vi "Agilent VNA Set Frequency On-Off.vi"(7 "Agilent VNA":T1, 8 "error in (no error)":errorcluster, 10 "Blank Frequencies (F)":bool, 11 "VISA Resource Name":refnum<visa-resource-name>) -> (0 "error out":errorcluster, 3 "dup VISA Resource Name":refnum<visa-resource-name>)   [LabVIEW 2011]
doc: "This VI for the HP8753B Network Analyzers reads the stimulus values. Except when performing log sweeps and freq list sweeps, this VI uses the start and stop values and the number of points to calcuate the stimulus values."
uses:
  TypeDefs/Agilent VNA Instrument Info.ctl
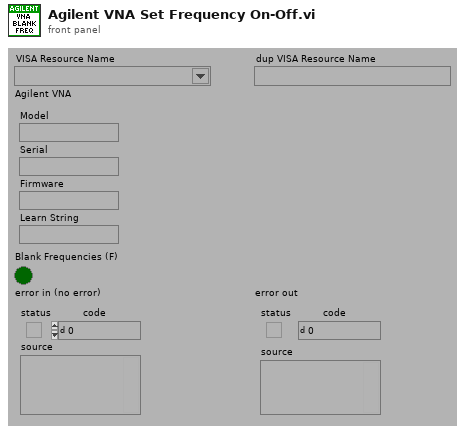
[diagram p1: front panel]
types:
  T1 = typedef "Agilent VNA Instrument Info.ctl" = cluster{"Model":string, "Serial":string, "Firmware":string, "Learn String":string}
  T2 = typedef "Agilent VNA Model.ctl" = enum16{"Not Supported", "8510X", "8719X", "8720X", "8722X", "8753X", "ENA", "PNA", "Field Fox"}
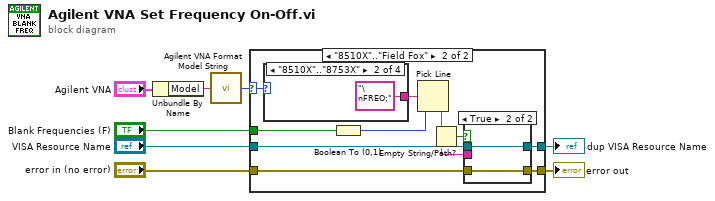
[diagram p0: block diagram]
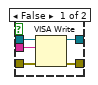
[diagram p3: hidden frame]
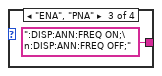
[diagram p5: hidden frame]
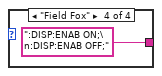
[diagram p6: hidden frame]
diagram:
  n1 = Unbundle By Name("Agilent VNA") -> ("Model"=w2:string)
  n2 = call "Agilent VNA Format Model String.vi"("Model"=w2) -> ("Model"=w1:T2)
  n3 = case shown="\"8510X\"..\"Field Fox\"" w1 {
    selector: w1 -> [_ w16]
    tunnel: [w10 w20] -> w8
    tunnel: [w9 w19] -> w7
    tunnel: "error in (no error)" -> [w9 w18]
    tunnel: "VISA Resource Name" -> [w10 w17]
    tunnel: "Blank Frequencies (F)" -> [_ w15]
    frame "Not Supported" {
    }
    frame "8510X".."Field Fox" {
      n4 = case shown="\"8510X\"..\"8753X\"" w16 {
        tunnel: [_ "\nFREO;" ":DISP:ANN:FREQ ON;\n:DISP:ANN:FREQ OFF;" ":DISP:ENAB ON;\n:DISP:ENAB OFF;"] -> w13
        frame "Not Supported" {
        }
        frame "8510X".."8753X" {
        }
        frame "ENA", "PNA" {
        }
        frame "Field Fox" {
        }
      }
      n5 = Boolean To (0,1)(Boolean=w15) -> (0, 1=w14:i16)
      n6 = Pick Line(multi-line string=w13, line index=w14) -> (output string=w12:string)  [unwired: 1 in]
      n7 = Empty String/Path?(string/path=w12) -> (empty?=w11:bool)
      n8 = case shown="True" w11 {
        tunnel: [w25 w27] -> w20
        tunnel: [w24 w26] -> w19
        tunnel: w18 -> [w23 w26]
        tunnel: w17 -> [w22 w27]
        tunnel: w12 -> [w21 _]
        frame False {
          n9 = VISA Write(VISA resource name=w22, write buffer=w21, error in (no error)=w23) -> (VISA resource name out=w25:refnum<visa-resource-name>, error out=w24:errorcluster)  [unwired: 1 out]
        }
        frame True {
        }
      }
    }
  }
  "dup VISA Resource Name" <- w8
  "error out" <- w7
